vi "Init.vi"(7 "Prepend Result Name":bool, 8 "error in (no error)":errorcluster, 9 "SA Pin":string, 10 "Measurement Name":string) -> (0 "error out":errorcluster, 3 "LTE_ACP out":refnum<class "LTE_ACP.lvclass">)   [LabVIEW 2016, in "SeqAuto Evaluations.lvlib" / "LTE_ACP.lvclass"]
uses:
  LTE_ACP.lvclass
  C:/Sequence Automation/Plugins/SeqAuto IEvaluation.lvlibp/SeqAuto IEvaluation.lvclass
  LTE_ACP.lvclass/LTE_ACP.ctl
  Private Methods/Write SA Pin.vi
  Plugins/SeqAuto IEvaluation.lvlibp/Write Measurement Name.vi
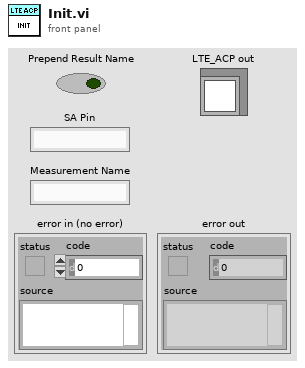
[diagram p1: front panel]
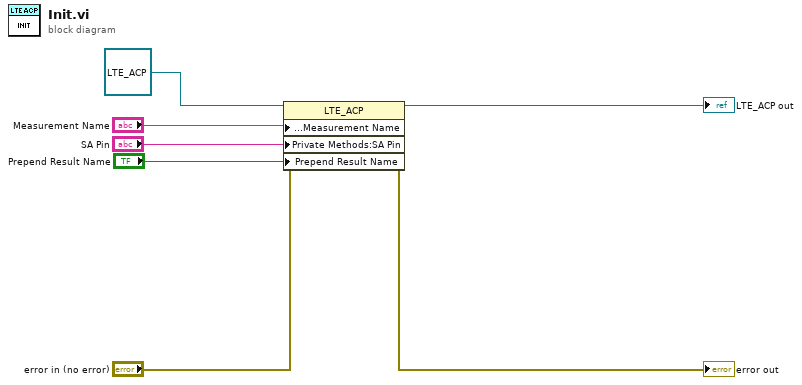
[diagram p0: block diagram]
diagram:
  n1 = property class="LTE_ACP"(reference=refnum<class "LTE_ACP.lvclass"> refnum ("LTE_ACP in"), error in="error in (no error)", "Protected Methods:Measurement Name"="Measurement Name", "Private Methods:SA Pin"="SA Pin", "Prepend Result Name"="Prepend Result Name") -> (reference out=→"LTE_ACP out":refnum<class "LTE_ACP.lvclass">, error out=→"error out":errorcluster)
